vi "Initialize HW.vi"(8 "error in (no error)":errorcluster, 11 "Simulated Servo in":refnum<class "Simulated Servo.lvclass">) -> (0 "error out":errorcluster, 3 "Simulated Servo out":refnum<class "Simulated Servo.lvclass">)   [LabVIEW 2020, in "Simulated Servo.lvclass"]
uses:
  Simulated Servo.lvclass
  Servo.lvclass
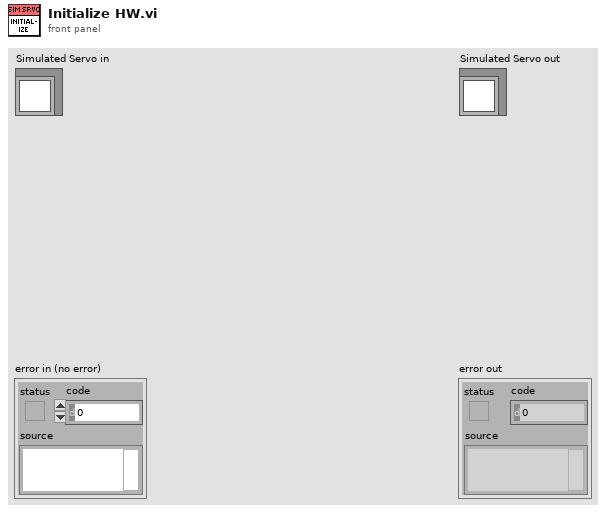
[diagram p1: front panel]
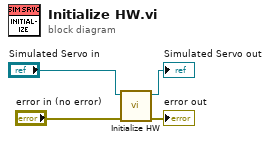
[diagram p0: block diagram]
diagram:
  n1 = call-parent "Initialize HW.vi"("error in (no error)"="error in (no error)", "Servo in"="Simulated Servo in") -> ("error out"=→"error out":errorcluster, "Servo out"=→"Simulated Servo out":refnum<class "Simulated Servo.lvclass">)  [unwired: 8 in]
